vi "Controls.vi"() -> ()   [LabVIEW 2017]
panel:
  out "Check Sensor":bool
  out "Check Hub":bool
  out "HUB ON":bool
  out "Inside °C":string
  in  "Auto Temp":bool
  in  "Adjust Temp":dbl
  in  "T ON/OFF":bool
  out "Outside °C":string
  out "Low Temp":bool
  out "Med Temp":bool
  out "High Temp":bool
  out "Cooler ON":bool
  out "Heater ON":bool
  out "Smoke Detected":bool
  in  "S ON/OFF":bool
  out "Smoke Meter":dbl(knob) scale=0.0..15.0
  out "Gas Detected":bool
  in  "G ON/OFF":bool
  out "LPG Gas Meter":dbl(knob) scale=0.0..10.0 scale format="%#_10g"
  # "CONTROLS"
  # "Illo inc."
  # "Temperaure Control System"
  # "Smoke Control System"
  # "Gas Control System"
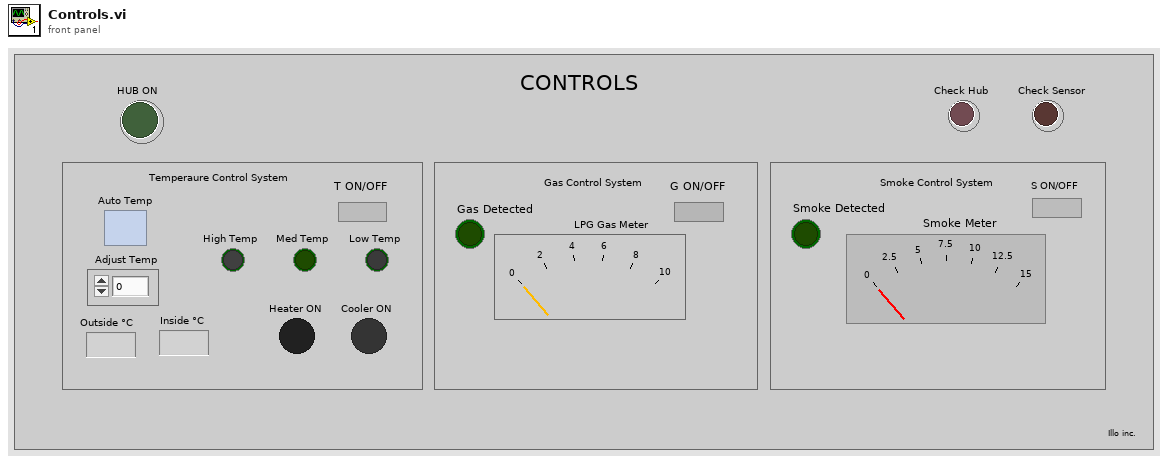
[diagram p1: front panel]
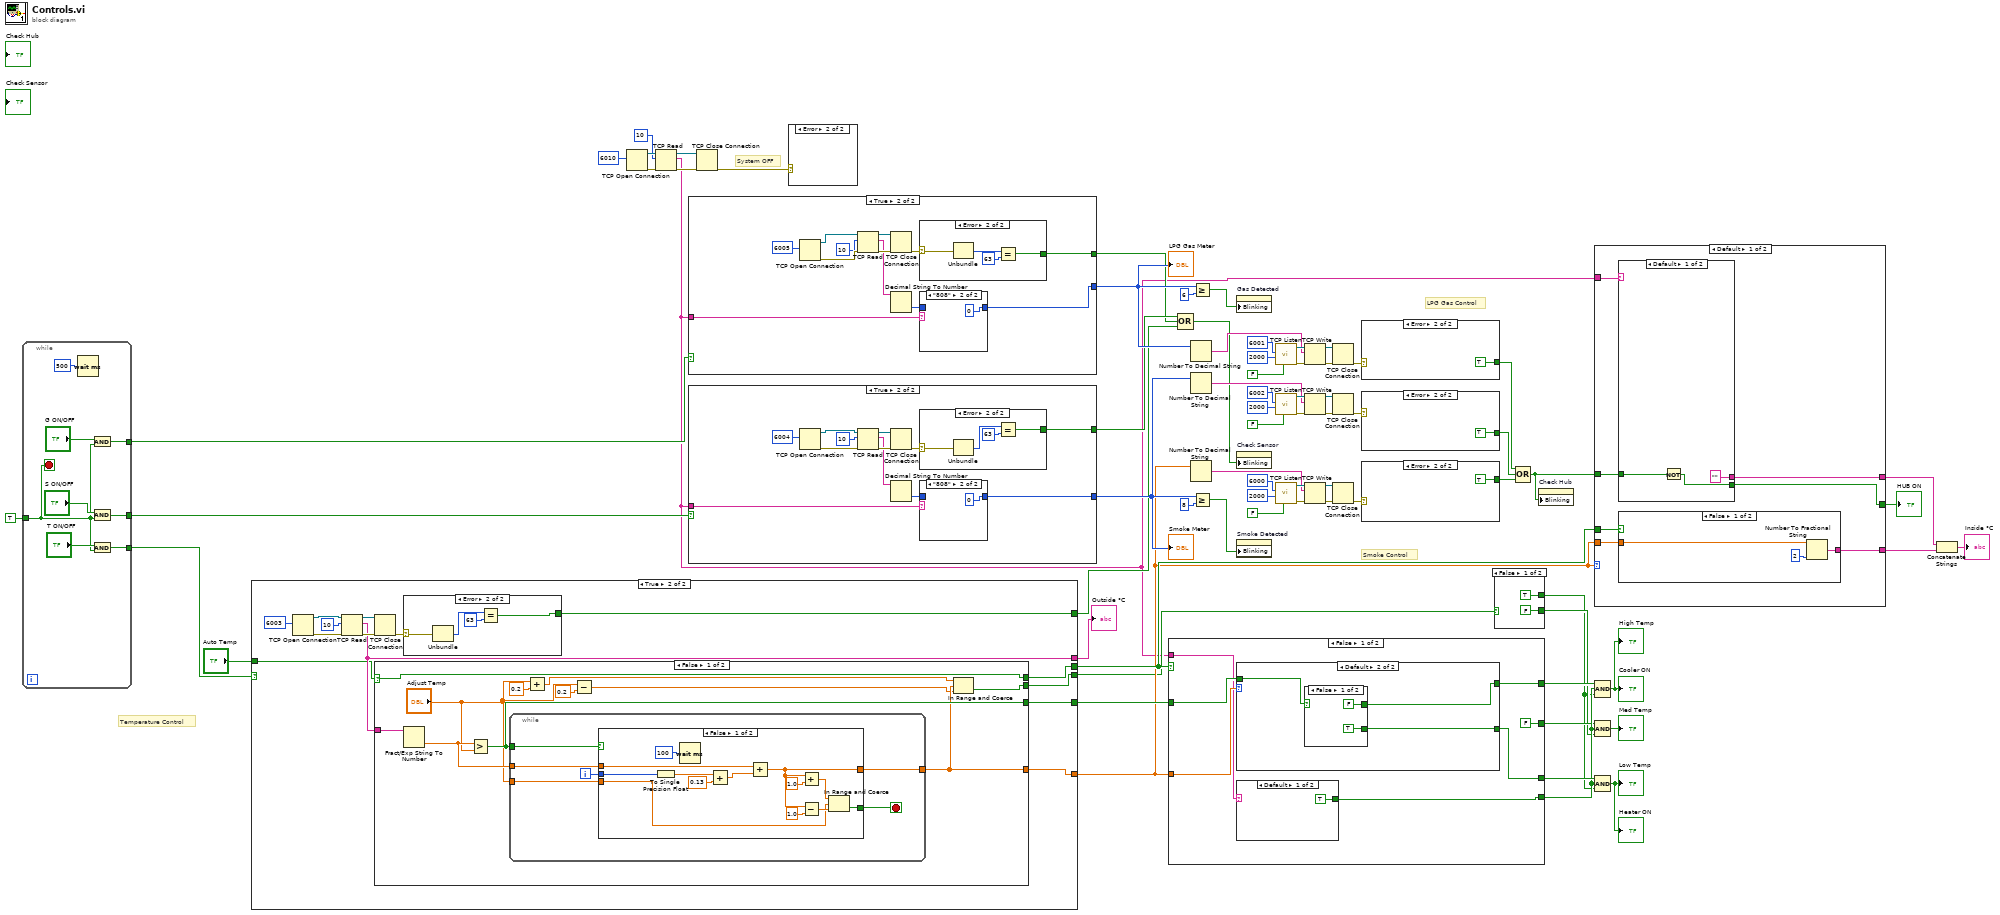
[diagram p0: block diagram]
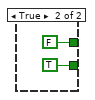
[diagram p2: hidden frame]
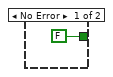
[diagram p4: hidden frame]
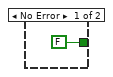
[diagram p5: hidden frame]
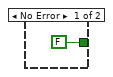
[diagram p6: hidden frame]
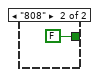
[diagram p7: hidden frame]
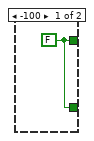
[diagram p8: hidden frame]
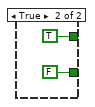
[diagram p9: hidden frame]
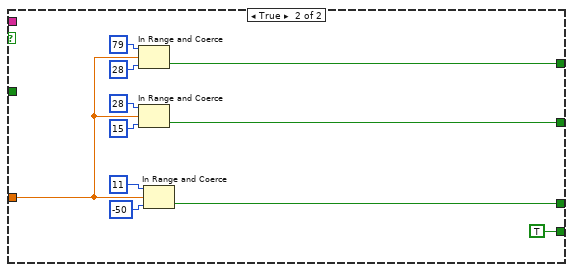
[diagram p10: hidden frame]
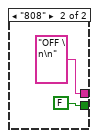
[diagram p11: hidden frame]
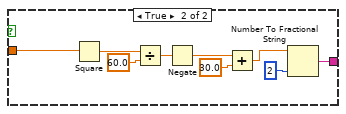
[diagram p12: hidden frame]
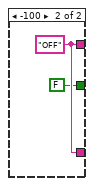
[diagram p13: hidden frame]
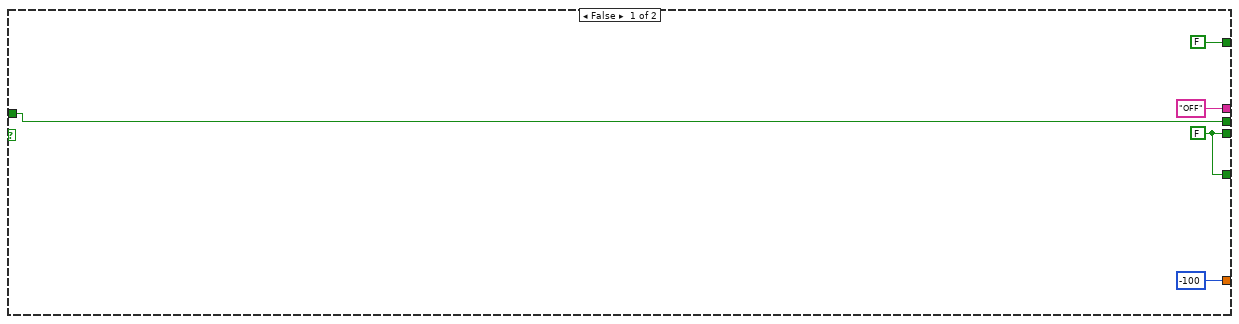
[diagram p14: hidden frame]
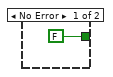
[diagram p15: hidden frame]
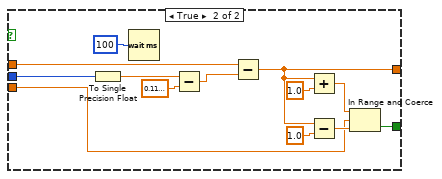
[diagram p16: hidden frame]
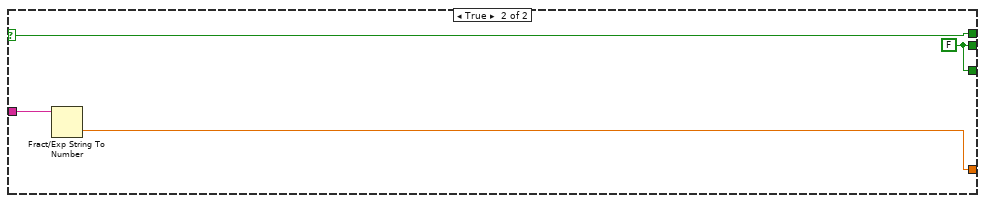
[diagram p17: hidden frame]
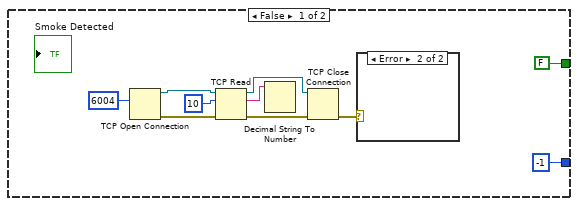
[diagram p18: hidden frame]
diagram:
  # "System OFF"
  # "Smoke Control"
  # "LPG Gas Control"
  # "Temperature Control"
  n1 = while {
    tunnel: TRUE -> [w73]
    tunnel: [w78] -> w45
    tunnel: [w75] -> w43
    tunnel: [w74] -> w41
    stop <- w73 stop-if-true
    n2 = Wait (ms)(milliseconds to wait=500) -> ()  [unwired: 1 out]
    n3 = And(x="G ON/OFF", y=w73) -> (x .and. y?=w78:bool)
    n4 = And(x="S ON/OFF", y=w73) -> (x .and. y?=w75:bool)
    n5 = And(x="T ON/OFF", y=w73) -> (x .and. y?=w74:bool)
  }
  n6 = case shown="True" w41 {
    tunnel: [-100 w99] -> w34
    tunnel: ["OFF" w91] -> w40
    tunnel: [w83 w90] -> w36
    tunnel: "Auto Temp" -> [w83 w89]
    tunnel: [w82 w88] -> w35
    tunnel: [w82 w87] -> w14
    tunnel: [FALSE w86] -> w5
    frame False {
      w82 = FALSE
    }
    frame True {
      n7 = TCP Open Connection(remote port or service name=6003) -> (connection ID=w95:refnum<k5>, error out=w94:errorcluster)  [unwired: 4 in]
      n8 = TCP Read(connection ID=w95, bytes to read=10, error in (no error)=w94) -> (connection ID out=w97:refnum<k5>, data out=w91:string, error out=w96:errorcluster)  [unwired: 2 in]
      n9 = TCP Close Connection(connection ID=w97, error in (no error)=w96) -> (error out=w98:errorcluster)  [unwired: 1 in, 1 out]
      n10 = case shown="False" w89 {
        selector: w89 -> [w113 w149]
        tunnel: [w109 w150] -> w99
        tunnel: w91 -> [w115 w151]
        tunnel: [w113 w149] -> w90
        tunnel: [w112 w148] -> w88
        tunnel: [w106 w148] -> w87
        frame False {
          n11 = Fract/Exp String To Number(string=w115) -> (number=w114:dbl)  [unwired: 3 in, 1 out]
          n12 = Greater?(x=w114, y="Adjust Temp") -> (0:w112:bool)
          n13 = while {
            tunnel: w114 -> [w121]
            tunnel: "Adjust Temp" -> [w120]
            tunnel: w112 -> [w118]
            tunnel: [w116] -> w109
            i -> [w119]
            stop <- w117 stop-if-true
            n14 = case shown="False" w118 {
              tunnel: w121 -> [w127 w140]
              tunnel: w120 -> [w128 w142]
              tunnel: w119 -> [w125 w138]
              tunnel: [w126 w139] -> w116
              tunnel: [w129 w141] -> w117
              frame False {
                n15 = To Single Precision Float(number=w125) -> (single precision float=w123:sgl)
                n16 = Wait (ms)(milliseconds to wait=u32 100) -> ()  [unwired: 1 out]
                n17 = Add(x=w123, y=0.13) -> (x+y=w122:dbl)
                n18 = Add(x=w127, y=w122) -> (x+y=w126:dbl)
                n19 = Add(x=w126, y=1.0) -> (x+y=w133:dbl)
                n20 = Subtract(x=w126, y=1.0) -> (x-y=w131:dbl)
                n21 = In Range and Coerce(upper limit=w133, x=w128, lower limit=w131) -> (In Range?=w129:bool)  [unwired: 1 out]
              }
              frame True {
                n22 = To Single Precision Float(number=w138) -> (single precision float=w137:sgl)
                n23 = Wait (ms)(milliseconds to wait=u32 100) -> ()  [unwired: 1 out]
                n24 = Subtract(x=w137, y=sgl 0.12) -> (x-y=w135:sgl)
                n25 = Subtract(x=w140, y=w135) -> (x-y=w139:dbl)
                n26 = Add(x=w139, y=1.0) -> (x+y=w146:dbl)
                n27 = Subtract(x=w139, y=1.0) -> (x-y=w144:dbl)
                n28 = In Range and Coerce(upper limit=w146, x=w142, lower limit=w144) -> (In Range?=w141:bool)  [unwired: 1 out]
              }
            }
          }
          n29 = Add(x="Adjust Temp", y=0.2 ("upper limit")) -> (x+y=w110:dbl)
          n30 = Subtract(x="Adjust Temp", y=0.2 ("lower limit")) -> (x-y=w107:dbl)
          n31 = In Range and Coerce(upper limit=w110, x=w109, lower limit=w107) -> (In Range?=w106:bool)  [unwired: 1 out]
        }
        frame True {
          w148 = FALSE
          n32 = Fract/Exp String To Number(string=w151) -> (number=w150:dbl)  [unwired: 3 in, 1 out]
        }
      }
      n33 = case shown="Error" w98 {
        selector: w98 -> [_ w104]
        tunnel: [FALSE w101] -> w86
        frame No Error {
        }
        frame Error {
          n34 = Unbundle(w104) -> ("code"=w103:i32)  [unwired: 2 out]
          n35 = Equal?(x=w103, y=63) -> (x = y?=w101:bool)
        }
      }
    }
  }
  "Outside °C" <- w40
  n36 = TCP Open Connection(remote port or service name=6010) -> (connection ID=w28:refnum<k5>, error out=w27:errorcluster)  [unwired: 4 in]
  n37 = TCP Read(connection ID=w28, bytes to read=10, error in (no error)=w27) -> (connection ID out=w30:refnum<k5>, data out=w1:string, error out=w29:errorcluster)  [unwired: 2 in]
  n38 = case shown="True" w45 {
    tunnel: [-1 w162] -> w44
    tunnel: [FALSE w165] -> w4
    tunnel: w1 -> [_ w164]
    frame False {
      n39 = TCP Open Connection(remote port or service name=6005) -> (connection ID=w158:refnum<k5>, error out=w157:errorcluster)  [unwired: 4 in]
      n40 = TCP Read(connection ID=w158, bytes to read=10, error in (no error)=w157) -> (connection ID out=w160:refnum<k5>, data out=w154:string, error out=w159:errorcluster)  [unwired: 2 in]
      n41 = Decimal String To Number(string=w154) -> ()  [unwired: 2 in, 2 out]
      n42 = TCP Close Connection(connection ID=w160, error in (no error)=w159) -> (error out=w153:errorcluster)  [unwired: 1 in, 1 out]
      n43 = case shown="Error" w153 {
        frame No Error {
        }
        frame Error {
        }
      }
    }
    frame True {
      n44 = TCP Open Connection(remote port or service name=6005) -> (connection ID=w171:refnum<k5>, error out=w170:errorcluster)  [unwired: 4 in]
      n45 = TCP Read(connection ID=w171, bytes to read=10, error in (no error)=w170) -> (connection ID out=w173:refnum<k5>, data out=w167:string, error out=w172:errorcluster)  [unwired: 2 in]
      n46 = TCP Close Connection(connection ID=w173, error in (no error)=w172) -> (error out=w166:errorcluster)  [unwired: 1 in, 1 out]
      n47 = Decimal String To Number(string=w167) -> (number=w163:i32)  [unwired: 2 in, 1 out]
      n48 = case shown="Error" w166 {
        selector: w166 -> [_ w178]
        tunnel: [FALSE w177] -> w165
        frame No Error {
        }
        frame Error {
          n49 = Unbundle(w178) -> ("code"=w180:i32)  [unwired: 2 out]
          n50 = Equal?(x=w180, y=63) -> (x = y?=w177:bool)
        }
      }
      n51 = case shown="\"808\"" w164 {
        tunnel: w163 -> [w174 _]
        tunnel: [w174 0] -> w162
        frame Default {
        }
        frame "808" {
        }
      }
    }
  }
  "LPG Gas Meter" <- w44
  n52 = case shown="True" w43 {
    tunnel: [-1 w191] -> w42
    tunnel: [FALSE w194] -> w6
    tunnel: w1 -> [_ w193]
    frame False {
      n53 = TCP Open Connection(remote port or service name=6004) -> (connection ID=w187:refnum<k5>, error out=w186:errorcluster)  [unwired: 4 in]
      n54 = TCP Read(connection ID=w187, bytes to read=10, error in (no error)=w186) -> (connection ID out=w189:refnum<k5>, data out=w183:string, error out=w188:errorcluster)  [unwired: 2 in]
      n55 = Decimal String To Number(string=w183) -> ()  [unwired: 2 in, 2 out]
      n56 = TCP Close Connection(connection ID=w189, error in (no error)=w188) -> (error out=w182:errorcluster)  [unwired: 1 in, 1 out]
      n57 = case shown="Error" w182 {
        frame No Error {
        }
        frame Error {
        }
      }
    }
    frame True {
      n58 = TCP Open Connection(remote port or service name=6004) -> (connection ID=w200:refnum<k5>, error out=w199:errorcluster)  [unwired: 4 in]
      n59 = TCP Read(connection ID=w200, bytes to read=10, error in (no error)=w199) -> (connection ID out=w202:refnum<k5>, data out=w196:string, error out=w201:errorcluster)  [unwired: 2 in]
      n60 = TCP Close Connection(connection ID=w202, error in (no error)=w201) -> (error out=w195:errorcluster)  [unwired: 1 in, 1 out]
      n61 = Decimal String To Number(string=w196) -> (number=w192:i32)  [unwired: 2 in, 1 out]
      n62 = case shown="Error" w195 {
        selector: w195 -> [_ w207]
        tunnel: [FALSE w206] -> w194
        frame No Error {
        }
        frame Error {
          n63 = Unbundle(w207) -> ("code"=w209:i32)  [unwired: 2 out]
          n64 = Equal?(x=w209, y=63) -> (x = y?=w206:bool)
        }
      }
      n65 = case shown="\"808\"" w193 {
        tunnel: [w203 0] -> w191
        tunnel: w192 -> [w203 _]
        frame Default {
        }
        frame "808" {
        }
      }
    }
  }
  "Smoke Meter" <- w42
  n66 = TCP Close Connection(connection ID=w30, error in (no error)=w29) -> (error out=w31:errorcluster)  [unwired: 1 in, 1 out]
  n67 = case shown="Error" w31 {
    frame No Error {
    }
    frame Error {
    }
  }
  n68 = case shown="False" w36 {
    tunnel: w34 -> [w212 w231]
    tunnel: [w214 w230] -> w24
    tunnel: [FALSE w229] -> w21
    tunnel: [w215 w228] -> w20
    tunnel: w35 -> [w216 _]
    tunnel: w1 -> [w211 _]
    tunnel: [w210 TRUE] -> w22
    frame False {
      n69 = case shown="Default" w212 {
        tunnel: w216 -> [_ w222]
        tunnel: [w219 w221] -> w215
        tunnel: [w219 w220] -> w214
        frame -100 {
          w219 = FALSE
        }
        frame Default {
          n70 = case shown="False" w222 {
            tunnel: [FALSE TRUE] -> w221
            tunnel: [TRUE FALSE] -> w220
            frame False {
            }
            frame True {
            }
          }
        }
      }
      n71 = case shown="Default" w211 {
        tunnel: [TRUE FALSE] -> w210
        frame Default {
        }
        frame "808" {
        }
      }
    }
    frame True {
      n72 = In Range and Coerce(upper limit=79, x=w231, lower limit=28) -> (In Range?=w228:bool)  [unwired: 1 out]
      n73 = In Range and Coerce(upper limit=28, x=w231, lower limit=15) -> (In Range?=w229:bool)  [unwired: 1 out]
      n74 = In Range and Coerce(upper limit=11, x=w231, lower limit=-50) -> (In Range?=w230:bool)  [unwired: 1 out]
    }
  }
  n75 = Compound Arithmetic op=OR(w6, w4, w5) -> (w7:bool)
  n76 = Number To Decimal String(number=w44) -> (decimal integer string=w57:string)  [unwired: 1 in]
  n77 = Number To Decimal String(number=w42) -> (decimal integer string=w50:string)  [unwired: 1 in]
  n78 = Number To Decimal String(number=w34) -> (decimal integer string=w65:string)  [unwired: 1 in]
  n79 = Greater Or Equal?(x=w44, y=6) -> (x >= y?=w39:bool)
  n80 = Greater Or Equal?(x=w42, y=8) -> (x >= y?=w38:bool)
  n81 = property on="Gas Detected" class="Bool (strict)"("Blinking"=w39) -> ()  [unwired: 2 in, 2 out]
  n82 = property on="Check Sensor" class="Bool (strict)"("Blinking"=w7) -> ()  [unwired: 2 in, 2 out]
  n83 = property on="Smoke Detected" class="Bool (strict)"("Blinking"=w38) -> ()  [unwired: 2 in, 2 out]
  n84 = call <vilib>:"TCP Listen.vi"("resolve remote address (T)"=FALSE, "timeout ms (wait forever: -1)"=2000, "port"=6001) -> ("error out"=w62:errorcluster, "connection ID"=w60:refnum<k5>)  [unwired: 4 in, 3 out]
  n85 = call <vilib>:"TCP Listen.vi"("resolve remote address (T)"=FALSE, "timeout ms (wait forever: -1)"=2000, "port"=6002) -> ("error out"=w55:errorcluster, "connection ID"=w53:refnum<k5>)  [unwired: 4 in, 3 out]
  n86 = call <vilib>:"TCP Listen.vi"("resolve remote address (T)"=FALSE, "timeout ms (wait forever: -1)"=2000, "port"=6000) -> ("error out"=w70:errorcluster, "connection ID"=w68:refnum<k5>)  [unwired: 4 in, 3 out]
  n87 = TCP Write(connection ID=w60, data in=w57, error in (no error)=w62) -> (connection ID out=w59:refnum<k5>, error out=w61:errorcluster)  [unwired: 1 in, 1 out]
  n88 = TCP Write(connection ID=w53, data in=w50, error in (no error)=w55) -> (connection ID out=w52:refnum<k5>, error out=w54:errorcluster)  [unwired: 1 in, 1 out]
  n89 = TCP Write(connection ID=w68, data in=w65, error in (no error)=w70) -> (connection ID out=w67:refnum<k5>, error out=w69:errorcluster)  [unwired: 1 in, 1 out]
  n90 = TCP Close Connection(connection ID=w59, error in (no error)=w61) -> (error out=w33:errorcluster)  [unwired: 1 in, 1 out]
  n91 = TCP Close Connection(connection ID=w52, error in (no error)=w54) -> (error out=w3:errorcluster)  [unwired: 1 in, 1 out]
  n92 = TCP Close Connection(connection ID=w67, error in (no error)=w69) -> (error out=w32:errorcluster)  [unwired: 1 in, 1 out]
  n93 = case shown="Error" w33 {
    tunnel: [FALSE TRUE] -> w10
    frame No Error {
    }
    frame Error {
    }
  }
  n94 = case shown="Error" w3 {
    tunnel: [FALSE TRUE] -> w9
    frame No Error {
    }
    frame Error {
    }
  }
  n95 = case shown="Error" w32 {
    tunnel: [FALSE TRUE] -> w8
    frame No Error {
    }
    frame Error {
    }
  }
  n96 = case shown="False" w14 {
    tunnel: [TRUE FALSE] -> w12
    tunnel: [FALSE TRUE] -> w13
    frame False {
    }
    frame True {
    }
  }
  n97 = Compound Arithmetic op=OR(w10, w9, w8) -> (w2:bool)
  n98 = property on="Check Hub" class="Bool (strict)"("Blinking"=w2) -> ()  [unwired: 2 in, 2 out]
  n99 = case shown="Default" w34 {
    tunnel: [w254 w273] -> w15
    tunnel: w36 -> [w253 _]
    tunnel: w34 -> [w252 _]
    tunnel: w1 -> [w251 _]
    tunnel: [w250 w273] -> w16
    tunnel: [w249 FALSE] -> w11
    tunnel: w2 -> [w248 _]
    frame Default {
      n100 = case shown="Default" w251 {
        tunnel: ["" "OFF \n\n"] -> w250
        tunnel: [w255 FALSE] -> w249
        tunnel: w248 -> [w256 _]
        frame Default {
          n101 = Not(x=w256) -> (.not. x?=w255:bool)
        }
        frame "808" {
        }
      }
      n102 = case shown="False" w253 {
        tunnel: [w261 w271] -> w254
        tunnel: w252 -> [w262 w265]
        frame False {
          n103 = Number To Fractional String(number=w262, precision (6)=i16 2) -> (F-format string=w261:string)  [unwired: 2 in]
        }
        frame True {
          n104 = Square(x=w265) -> (x^2=w270:dbl)
          n105 = Divide(x=w270, y=60.0) -> (x/y=w267:dbl)
          n106 = Negate(x=w267) -> (-x=w266:dbl)
          n107 = Add(x=w266, y=30.0) -> (x+y=w264:dbl)
          n108 = Number To Fractional String(number=w264, precision (6)=i16 2) -> (F-format string=w271:string)  [unwired: 2 in]
        }
      }
    }
    frame -100 {
      w273 = "OFF"
    }
  }
  "HUB ON" <- w11
  n109 = Compound Arithmetic op=AND(w20, w22, w12) -> (→"Cooler ON" →"High Temp":bool)
  n110 = Compound Arithmetic op=AND(w21, w22, w13) -> (→"Med Temp":bool)
  n111 = Compound Arithmetic op=AND(w24, w22, w12) -> (→"Heater ON" →"Low Temp":bool)
  n112 = Concatenate Strings(w16, w15) -> (→"Inside °C":string)
